vi "Camera Performance.vi"() -> ()   [LabVIEW 2013]
uses:
  <vilib>/Rock Robotics/WPI/Camera/WPI_CameraFrameRate.ctl
  <vilib>/Rock Robotics/WPI/Camera/WPI_CameraImageSize.ctl
  <vilib>/Rock Robotics/WPI/Camera/WPI_CameraExposure Priority Values.ctl
  <vilib>/Rock Robotics/WPI/Camera/WPI_CameraExposure Values.ctl
  <vilib>/Rock Robotics/WPI/Camera/WPI_CameraWhite Balance Values.ctl
panel:
  in  "Display":bool
  in  "Color Enabled":bool=TRUE
  in  "MJPG":bool=TRUE
  in  "White Balance":T1
  in  "Exposure":T2
  in  "Color Level":i32=50 min=0 max=100
  in  "Exposure Priority":T3
  in  "Sharpness":i32=50 min=0 max=100
  in  "Brightness":i32=50 min=0 max=100
  in  "Compression":i32=30
  in  "Image Size":T4=enum."320x240"
  in  "Frame Rate (fps)":T5=30 min=1 max=30
  in  "stop":bool
  out "Waveform Chart":u32(graph)
  out "Image":T6(plugin-control)
  # "Before running the VI, select between\nMJPG and JPG .\nYou can change all other camera settings\nwhile the program runs to view the\nperformance tradeoffs."
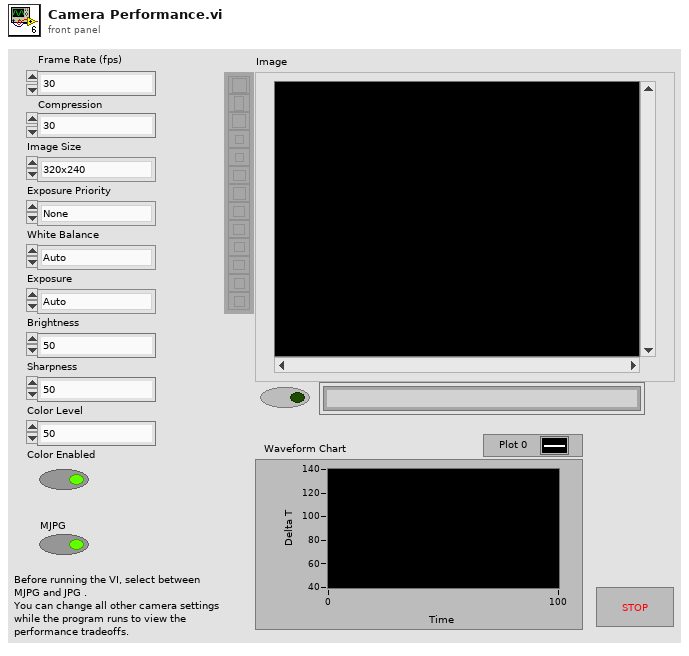
[diagram p1: front panel]
types:
  T1 = typedef "WPI_CameraWhite Balance Values.ctl" = enum16{"Auto", "Fixed indoor", "Fixed outdoor 1", "Fixed outdoor 2", "Fixed fluorescent 1", "Fixed fluorescent 2", "Hold current"}
  T2 = typedef "WPI_CameraExposure Values.ctl" = enum16{"Auto", "Flicker-free 50 Hz", "Flicker-free 60 Hz", "Hold current"}
  T3 = typedef "WPI_CameraExposure Priority Values.ctl" = enum16{"None", "Prioritize frame rate", "Prioritize image quality"}
  T4 = typedef "WPI_CameraImageSize.ctl" = enum16{"640x480", "320x240", "160x120"}
  T5 = typedef "WPI_CameraFrameRate.ctl" = u32
  T6 = typedef "IMAQ Image.ctl" = refnum<image>
  T7 = typedef "Image Type" = u32
  T8 = typedef "WPI_CameraDevRef.ctl" = cluster{"Camera Address":string, "CameraStatus":errorcluster, "Acquire Image Notifier":refnum<notifier>}
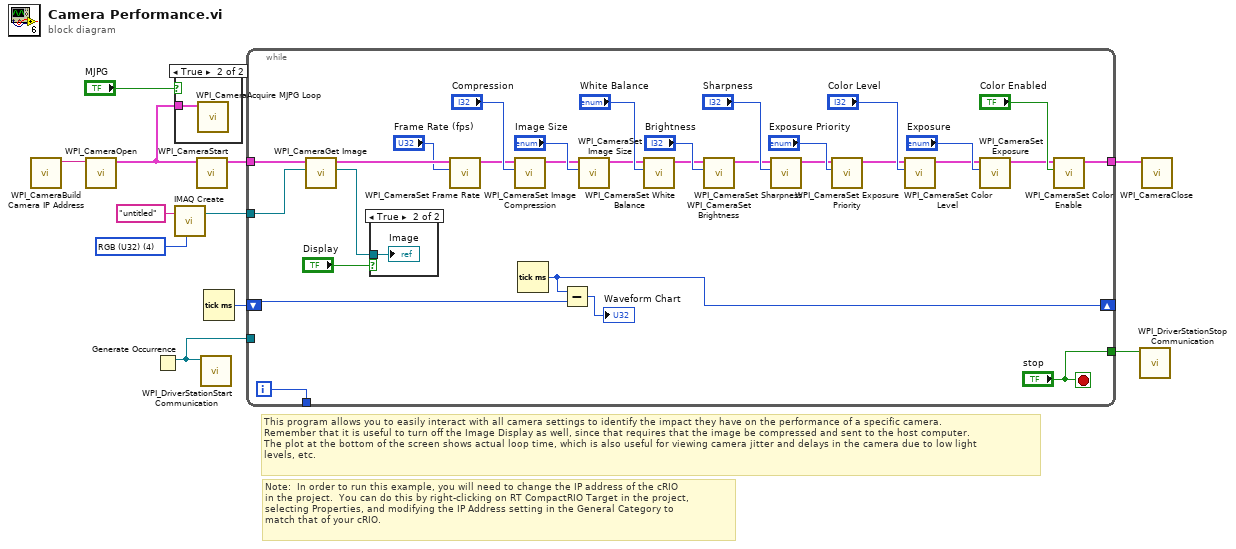
[diagram p0: block diagram]
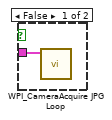
[diagram p2: hidden frame]
diagram:
  w9 = T7 4 items=["Grayscale (U8)", "Grayscale (I16)", "Grayscale (SGL)", "Complex (CSG)", "RGB (U32)", "HSL (U32)", "RGB (U64)", "Grayscale (U16)"] ("Image Type")
  # "Note:  In order to run this example, you will need to change the IP address of the cRIO\nin the project.  You can do this by right-clicking on RT CompactRIO Target in the project,\nselecting Properties, and modifying the IP Address setting in the General Category to \nmatch that of your cRIO."
  # "This program allows you to easily interact with all camera settings to identify the impact they have on the performance of a specific camera.\nRemember that it is useful to turn off the Image Display as well, since that requires that the image be compressed and sent to the host computer.\nThe plot at the bottom of the screen shows actual loop time, which is also useful for viewing camera jitter and delays in the camera due to low light\nlevels, etc."
  n1 = call <vilib>:"WPI_CameraBuild Camera IP Address.vi"() -> ("Camera Address"=w2:string)  [unwired: 11 in]
  n2 = call <vilib>:"WPI_CameraOpen.vi"("Camera Address"=w2) -> ("CameraDevRef"=w5:T8)  [unwired: 9 in, 1 out]
  n3 = Generate Occurrence() -> (w3:refnum<k4>)
  n4 = case shown="True" "MJPG" {
    tunnel: w5 -> [w12 w13]
    frame False {
      n5 = call <vilib>:"WPI_CameraAcquire JPG Loop.vi"("CameraDevRef"=w12) -> ()  [unwired: 11 in]
    }
    frame True {
      n6 = call <vilib>:"WPI_CameraAcquire MJPG Loop.vi"("CameraDevRef"=w13) -> ()  [unwired: 11 in]
    }
  }
  n7 = call "IMAQ Create"("Image Name"="untitled", "Image Type"=w9) -> ("New Image"=w11:T6)  [unwired: 3 in, 1 out]
  n8 = call <vilib>:"WPI_CameraStart.vi"("CameraDevRef"=w5) -> ("CameraDevRef Out"=w8:T8)  [unwired: 9 in, 1 out]
  n9 = call <vilib>:"WPI_DriverStationStart Communication.vi"("occurrence"=w3) -> ()  [unwired: 11 in]
  n10 = Tick Count (ms)() -> (millisecond timer value=w7:u32)
  n11 = while {
    tunnel: w8 -> [w43]
    tunnel: w11 -> [w42]
    shift-right: [w39] -> _
    shift-left: w7 -> [w40]
    tunnel: [w36] -> w6
    tunnel: [w16] -> _
    tunnel: w3 -> [_]
    tunnel: ["stop"] -> w1
    i -> [w16]
    stop <- "stop" stop-if-true
    n12 = call <vilib>:"WPI_CameraGet Image.vi"("Image"=w42, "CameraDevRef"=w43) -> ("Image Out"=w41:T6, "CameraDevRef Out"=w37:T8)  [unwired: 7 in, 1 out]
    n13 = case shown="True" "Display" {
      tunnel: w41 -> [_ w44]
      frame False {
      }
      frame True {
        "Image" <- w44
      }
    }
    n14 = call <vilib>:"WPI_CameraSet Frame Rate.vi"("Frame Rate (fps)"="Frame Rate (fps)", "CameraDevRef"=w37) -> ("CameraDevRef Out"=w25:T8)  [unwired: 8 in, 1 out]
    n15 = call <vilib>:"WPI_CameraSet Image Compression.vi"("Compression"="Compression", "CameraDevRef"=w25) -> ("CameraDevRef Out"=w24:T8)  [unwired: 8 in, 1 out]
    n16 = Tick Count (ms)() -> (millisecond timer value=w39:u32)
    n17 = Subtract(x=w39, y=w40) -> (x-y=→"Waveform Chart":u32)
    n18 = call <vilib>:"WPI_CameraSet Image Size.vi"("Image Size"="Image Size", "CameraDevRef"=w24) -> ("CameraDevRef Out"=w18:T8)  [unwired: 8 in, 1 out]
    n19 = call <vilib>:"WPI_CameraSet White Balance.vi"("White Balance"="White Balance", "CameraDevRef"=w18) -> ("CameraDevRef Out"=w23:T8)  [unwired: 8 in, 1 out]
    n20 = call <vilib>:"WPI_CameraSet Brightness.vi"("Brightness"="Brightness", "CameraDevRef"=w23) -> ("CameraDevRef Out"=w22:T8)  [unwired: 8 in, 1 out]
    n21 = call <vilib>:"WPI_CameraSet Sharpness.vi"("Sharpness"="Sharpness", "CameraDevRef"=w22) -> ("CameraDevRef Out"=w21:T8)  [unwired: 8 in, 1 out]
    n22 = call <vilib>:"WPI_CameraSet Exposure Priority.vi"("Exposure Priority"="Exposure Priority", "CameraDevRef"=w21) -> ("CameraDevRef Out"=w20:T8)  [unwired: 8 in, 1 out]
    n23 = call <vilib>:"WPI_CameraSet Color Level.vi"("Color Level"="Color Level", "CameraDevRef"=w20) -> ("CameraDevRef Out"=w19:T8)  [unwired: 8 in, 1 out]
    n24 = call <vilib>:"WPI_CameraSet Exposure.vi"("Exposure"="Exposure", "CameraDevRef"=w19) -> ("CameraDevRef Out"=w17:T8)  [unwired: 8 in, 1 out]
    n25 = call <vilib>:"WPI_CameraSet Color Enable.vi"("Color Enabled"="Color Enabled", "CameraDevRef"=w17) -> ("CameraDevRef Out"=w36:T8)  [unwired: 8 in, 1 out]
  }
  n26 = call <vilib>:"WPI_DriverStationStop Communication.vi"("StopCommunication"=w1) -> ()  [unwired: 1 in, 10 out]
  n27 = call <vilib>:"WPI_CameraClose.vi"("CameraDevRef"=w6) -> ()  [unwired: 10 in, 1 out]
